vi "Generate_WayPoints_Hopping_CV_RunningAvg.vi"(11 "Input Cluster":T2={"Scan Rate (um/s)"=15.0, "X Start"=15.0, "X End"=15.0, "Y Start"=15.0, "Y End"=15.0, " Z Start"=15.0, "HoppingDistance"=1.0, "V"=15.0, "Z End"=15.0, "Approach Rate Hopping (um/s)"=15.0, "Retrack Rate (um/s)"=15.0, "V 2"=15.0, "Approach Rate (um/s)"=15.0, "V 3"=15.0, "CV Rate / V/s"=15.0, "V 4"=15.0, "V 1"=15.0, "HoldTime1/s"=15.0, "Hold time 2 / s"=15.0, "Hold time 3/ s"=15.0, "V2 (AO4)Approach"=15.0, "V2 (AO4)CV"=15.0}) -> (0 "output cluster":T1)   [LabVIEW 2023]
uses:
  TypeDefs/WayPointCluster.ctl
  User_Vi/Settings.vi
panel:
  in  "WayPointCluster":T1
  out "Y  P":dbl
  out "X  P":dbl
  out "HoppingDistanceX":dbl
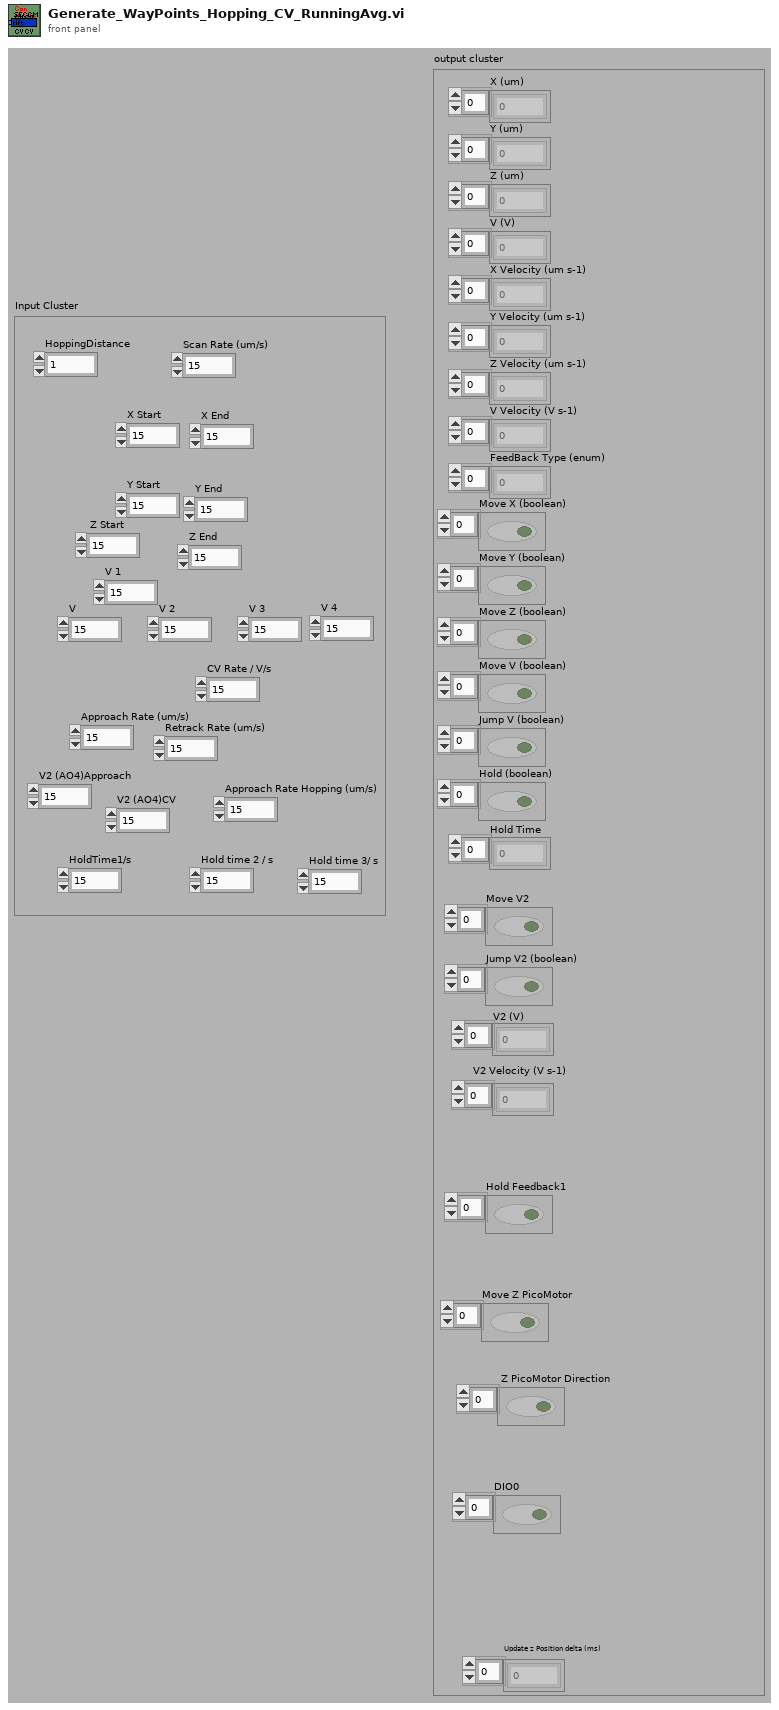
[diagram p1: front panel]
types:
  T1 = typedef "WayPointCluster.ctl" = cluster{"X (um)":dbl[], "Y (um)":dbl[], "Z (um)":dbl[], "V (V)":dbl[], "X Velocity (um s-1)":dbl[], "Y Velocity (um s-1)":dbl[], "Z Velocity (um s-1)":dbl[], "V Velocity (V s-1)":dbl[], "FeedBack Type (enum)":u16[], "Move X (boolean)":bool[], "Move Y (boolean)":bool[], "Move Z (boolean)":bool[], "Move V (boolean)":bool[], "Jump V (boolean)":bool[], "Hold (boolean)":bool[], "Hold Time":u32[], "V2 (V)":dbl[], "Move V2":bool[], "V2 Velocity (V s-1)":dbl[], "Jump V2 (boolean)":bool[], "Update z Position delta (ms)":i16[], "Hold Feedback1":bool[], "Move Z PicoMotor":bool[], " Z PicoMotor Direction":bool[], "DIO0":bool[]}
  T2 = cluster{"Scan Rate (um/s)":dbl, "X Start":dbl, "X End":dbl, "Y Start":dbl, "Y End":dbl, " Z Start":dbl, "HoppingDistance":dbl, "V":dbl, "Z End":dbl, "Approach Rate Hopping (um/s)":dbl, "Retrack Rate (um/s)":dbl, "V 2":dbl, "Approach Rate (um/s)":dbl, "V 3":dbl, "CV Rate / V/s":dbl, "V 4":dbl, "V 1":dbl, "HoldTime1/s":dbl, "Hold time 2 / s":dbl, "Hold time 3/ s":dbl, "V2 (AO4)Approach":dbl, "V2 (AO4)CV":dbl}
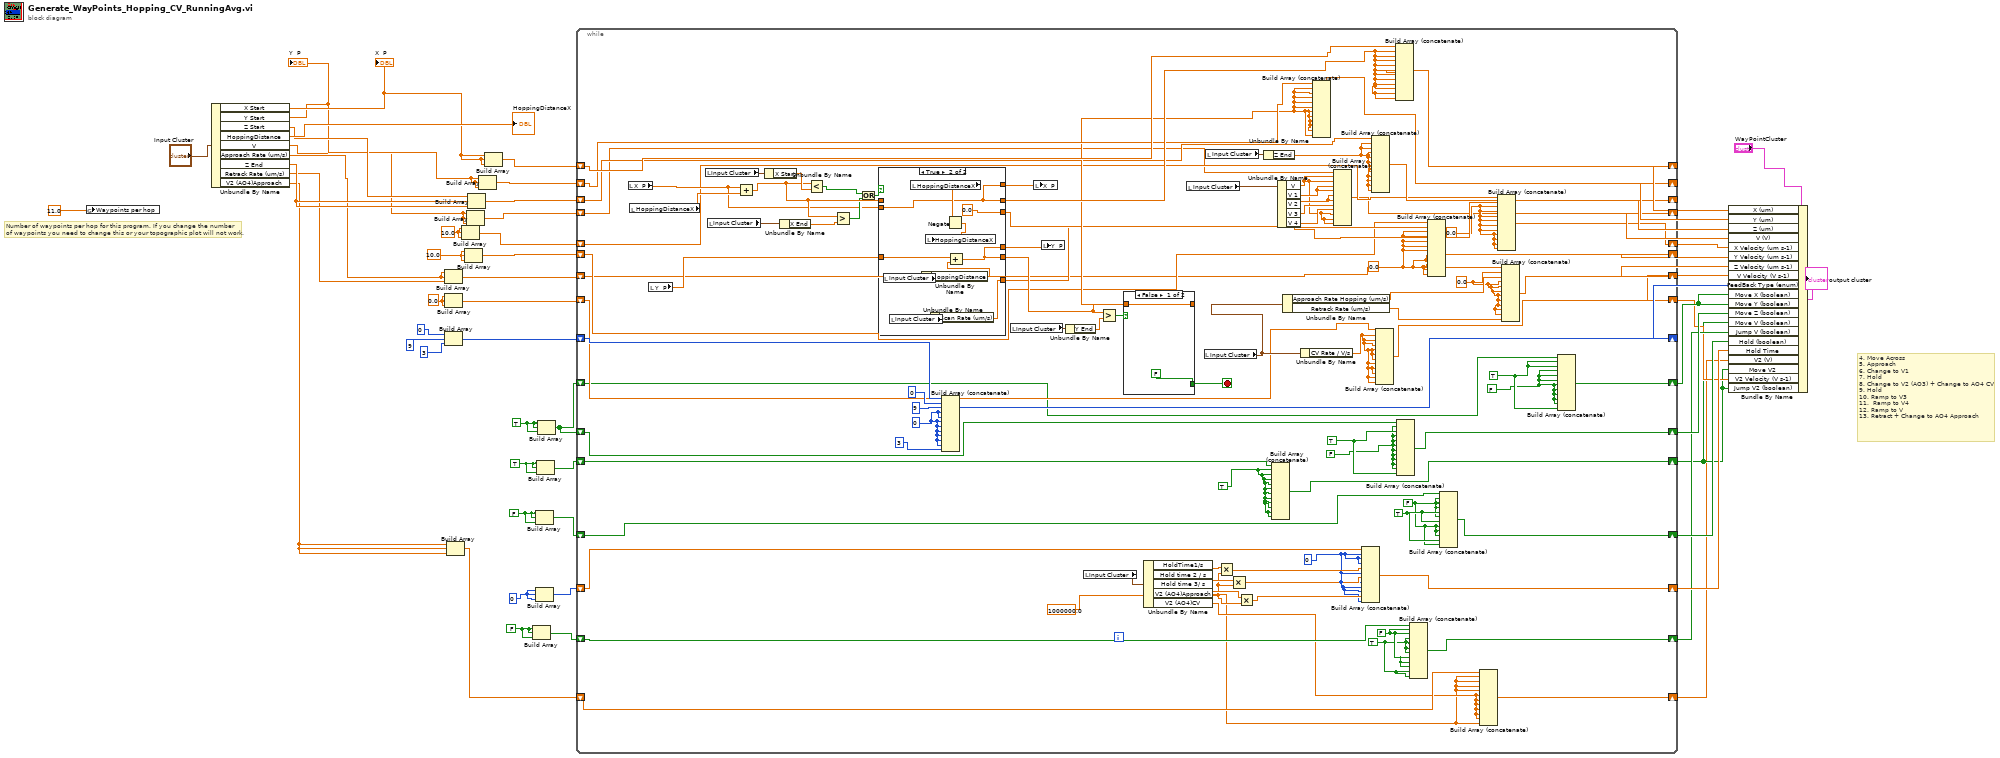
[diagram p0: block diagram]
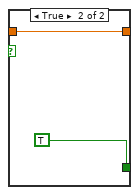
[diagram p2: hidden frame]
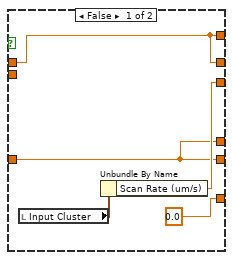
[diagram p3: hidden frame]
diagram:
  w17 = FALSE
  w20 = FALSE
  w19 = u32 0 ("element")
  w18 = TRUE
  w15 = TRUE
  w11 = 10.0 ("element")
  w12 = 10.0 ("element")
  w14 = 0.0 ("element")
  # "Number of waypoints per hop for this program. If you change the number\nof waypoints you need to change this or your topographic plot will not work."
  # "4. Move Across\n5. Approach\n6. Change to V1\n7. Hold\n8. Change to V2 (AO3) + Change to AO4 CV\n9. Hold\n10. Ramp to V3\n11.  Ramp to V4\n12. Ramp to V\n13. Retract + Change to AO4 Approach"
  n1 = global write "Settings.vi" "Waypoints per hop"(11.0) -> ()
  n2 = Unbundle By Name("Input Cluster") -> ("X Start"=w35:dbl, "Y Start"=w34:dbl, "Z Start"=w36:dbl, "HoppingDistance"=→"HoppingDistanceX":dbl, "V"=w32:dbl, "Approach Rate (um/s)"=w13:dbl, "Z End"=w33:dbl, "Retrack Rate (um/s)"=w31:dbl, "V2 (AO4)Approach"=w4:dbl)
  "X  P" <- w35
  "Y  P" <- w34
  n3 = Build Array(w13, w13, w31) -> (w42:dbl[])
  n4 = Build Array(u16 0 ("element"), u16 9 ("element"), u16 3 ("element")) -> (w39:u16[])
  n5 = Build Array(w14, w14, w14) -> (w40:dbl[])
  n6 = Build Array(w4, w4, w4) -> (w3:dbl[])
  n7 = Build Array(w11, w11, w11) -> (w45:dbl[])
  n8 = Build Array(w12, w12, w12) -> (w44:dbl[])
  n9 = Build Array(w32, w32, w32) -> (w47:dbl[])
  n10 = Build Array(w36, w33, w33) -> (w49:dbl[])
  n11 = Build Array(w34, w34, w34) -> (w51:dbl[])
  n12 = Build Array(w35, w35, w35) -> (w53:dbl[])
  n13 = Build Array(w20, w20, w20) -> (w24:bool[])
  n14 = Build Array(w17, w17, w17) -> (w16:bool[])
  n15 = Build Array(w19, w19, w19) -> (w28:u32[])
  n16 = Build Array(w18, w18, w18) -> (w22:bool[])
  n17 = Build Array(w15, w15, w15) -> (w7:bool[])
  n18 = while {
    shift-right: [w120] -> w52
    shift-left: w53 -> [w121]
    shift-right: [w117] -> w50
    shift-left: w51 -> [w118]
    shift-right: [w114] -> w48
    shift-left: w49 -> [w115]
    shift-right: [w104] -> w46
    shift-left: w47 -> [w105]
    shift-right: [w98] -> w29
    shift-left: w45 -> [w112]
    shift-right: [w107] -> w43
    shift-left: w44 -> [w108]
    shift-right: [w96] -> w41
    shift-left: w42 -> [w97]
    shift-right: [w91] -> w6
    shift-left: w40 -> [w92]
    shift-right: [w144] -> w38
    shift-left: w39 -> [w145]
    shift-right: [w88] -> w27
    shift-left: w7 -> [w89]
    shift-right: [w82] -> w26
    shift-left: w16 -> [w83]
    shift-right: [w78] -> w25
    shift-left: w28 -> [w79]
    shift-right: [w68] -> w23
    shift-left: w24 -> [w69]
    shift-right: [w85] -> w5
    shift-left: w22 -> [w86]
    shift-right: [w61] -> w8
    shift-left: w7 -> [w60]
    shift-right: [w58] -> w2
    shift-left: w3 -> [w59]
    stop <- w132 stop-if-true
    w63 = FALSE
    w64 = TRUE
    w65 = 1000000.0 ("y")
    w66 = TRUE
    w110 = 0.0 ("element")
    w84 = TRUE
    w67 = FALSE
    w70 = u32 0 ("element")
    w81 = TRUE
    w80 = FALSE
    w62 = FALSE
    w87 = TRUE
    w123 = u16 0 ("element")
    w106 = 0.0 ("element")
    w94 = 0.0 ("element")
    n19 = local read "X  P"() -> (w131:dbl)
    n20 = local read "HoppingDistanceX"() -> (w146:dbl)
    n21 = local read "Y  P"() -> (w130:dbl)
    n22 = local read "Input Cluster"() -> (w148:T2)
    n23 = local read "Input Cluster"() -> (w147:T2)
    n24 = Add(x=w131, y=w146) -> (x+y=w138:dbl)
    n25 = Unbundle By Name(w148) -> ("X Start"=w141:dbl)
    n26 = Unbundle By Name(w147) -> ("X End"=w139:dbl)
    n27 = Less?(x=w138, y=w141) -> (x < y?=w140:bool)
    n28 = Greater?(x=w138, y=w139) -> (0:w137:bool)
    n29 = Or(x=w140, y=w137) -> (x .or. y?=w136:bool)
    n30 = case shown="True" w136 {
      tunnel: w138 -> [w153 _]
      tunnel: [w153 w159] -> w119
      tunnel: w131 -> [_ w159]
      tunnel: w130 -> [w154 w160]
      tunnel: [w154 w158] -> w129
      tunnel: [w156 0.0] -> w111
      tunnel: [0.0 w161] -> w109
      tunnel: [w154 w158] -> w128
      tunnel: [w153 w159] -> w127
      frame False {
        n31 = local read "Input Cluster"() -> (w157:T2)
        n32 = Unbundle By Name(w157) -> ("Scan Rate (um/s)"=w156:dbl)
      }
      frame True {
        n33 = local read "Input Cluster"() -> (w165:T2)
        n34 = local read "Input Cluster"() -> (w163:T2)
        n35 = local read "HoppingDistanceX"() -> (w167:dbl)
        n36 = Unbundle By Name(w165) -> ("HoppingDistance"=w164:dbl)
        n37 = Unbundle By Name(w163) -> ("Scan Rate (um/s)"=w161:dbl)
        n38 = Negate(x=w167) -> (-x=w166:dbl)
        n39 = local write "HoppingDistanceX"(w166) -> ()
        n40 = Add(x=w160, y=w164) -> (x+y=w158:dbl)
      }
    }
    n41 = Build Array (concatenate)(w145, u16 0 ("element"), u16 9 ("element"), w123, w123, w123, w123, w123, w123, w123, w123, u16 3 ("element")) -> (w144:u16[])
    n42 = local read "Input Cluster"() -> (w135:T2)
    n43 = local write "X  P"(w127) -> ()
    n44 = local write "Y  P"(w128) -> ()
    n45 = Unbundle By Name(w135) -> ("Y End"=w134:dbl)
    n46 = local read "Input Cluster"() -> (w77:T2)
    n47 = Greater?(x=w129, y=w134) -> (0:w133:bool)
    n48 = case shown="False" w133 {
      tunnel: w129 -> [w150 w152]
      tunnel: [w150 w152] -> w116
      tunnel: [FALSE TRUE] -> w132
      frame False {
      }
      frame True {
      }
    }
    n49 = Unbundle By Name(w77) -> ("HoldTime1/s"=w76:dbl, "Hold time 2 / s"=w75:dbl, "Hold time 3/ s"=w74:dbl, "V2 (AO4)Approach"=w56:dbl, "V2 (AO4)CV"=w57:dbl)
    n50 = local read "Input Cluster"() -> (w142:T2)
    n51 = local read "Input Cluster"() -> (w124:T2)
    n52 = local read "Input Cluster"() -> (w143:T2)
    n53 = Multiply(x=w76, y=w65) -> (x*y=w73:dbl)
    n54 = Multiply(x=w75, y=w65) -> (x*y=w72:dbl)
    n55 = Multiply(x=w74, y=w65) -> (x*y=w71:dbl)
    n56 = Unbundle By Name(w143) -> ("Z End"=w113:dbl)
    n57 = Build Array (concatenate)(w86, w84, w84, w84, w84, w84, w84, w84, w84, w84, w84, w84) -> (w85:bool[])
    n58 = Unbundle By Name(w142) -> ("V"=w99:dbl, "V 1"=w103:dbl, "V 2"=w102:dbl, "V 3"=w101:dbl, "V 4"=w100:dbl)
    n59 = Unbundle By Name(w124) -> ("Approach Rate Hopping (um/s)"=w95:dbl, "Retrack Rate (um/s)"=w93:dbl)
    n60 = Unbundle By Name(w124) -> ("CV Rate / V/s"=w90:dbl)
    n61 = Build Array (concatenate)(w118, w116, w116, w116, w116, w116, w116, w116, w116, w116, w116, w116) -> (w117:dbl[])
    n62 = Build Array (concatenate)(w105, w99, w99, w103, w103, w102, w102, w101, w100, w99, w99, w99) -> (w104:dbl[])
    n63 = Build Array (concatenate)(w79, w70, w70, w70, w73, w70, w72, w70, w70, w70, w71, w70) -> (w78:dbl[])
    n64 = Build Array (concatenate)(w115, w113, w113, w113, w113, w113, w113, w113, w113, w113, w113, w113) -> (w114:dbl[])
    n65 = Build Array (concatenate)(w92, w90, w90, w90, w90, w90, w90, w90, w90, w90, w90, w90) -> (w91:dbl[])
    n66 = Build Array (concatenate)(w121, w119, w119, w119, w119, w119, w119, w119, w119, w119, w119, w119) -> (w120:dbl[])
    n67 = Build Array (concatenate)(w89, w62, w87, w62, w62, w62, w62, w62, w62, w62, w62, w87) -> (w88:bool[])
    n68 = Build Array (concatenate)(w69, w67, w67, w66, w66, w66, w66, w67, w67, w67, w66, w66) -> (w68:bool[])
    n69 = Build Array (concatenate)(w108, w109, w106, w106, w106, w106, w106, w106, w106, w106, w106, w106) -> (w107:dbl[])
    n70 = Build Array (concatenate)(w83, w80, w80, w80, w81, w80, w81, w80, w80, w80, w81, w80) -> (w82:bool[])
    n71 = Build Array (concatenate)(w59, w56, w56, w56, w56, w57, w57, w57, w57, w57, w57, w56) -> (w58:dbl[])
    n72 = Build Array (concatenate)(w112, w111, w110, w110, w110, w110, w110, w110, w110, w110, w110, w110) -> (w98:dbl[])
    n73 = Build Array (concatenate)(w97, w94, w95, w94, w94, w94, w94, w94, w94, w94, w94, w93) -> (w96:dbl[])
    n74 = Build Array (concatenate)(w60, w64, w64, w63, w63, w63, w63, w63, w63, w63, w63, w64) -> (w61:bool[])
  }
  n75 = Bundle By Name(cluster="WayPointCluster", "X (um)"=w52, "Y (um)"=w50, "Z (um)"=w48, "V (V)"=w46, "X Velocity (um s-1)"=w29, "Y Velocity (um s-1)"=w43, "Z Velocity (um s-1)"=w41, "V Velocity (V s-1)"=w6, "FeedBack Type (enum)"=w38, "Move X (boolean)"=w8, "Move Y (boolean)"=w8, "Move Z (boolean)"=w27, "Move V (boolean)"=w5, "Jump V (boolean)"=w23, "Hold (boolean)"=w26, "Hold Time"=w25, "V2 (V)"=w2, "Move V2"=w5, "V2 Velocity (V s-1)"=w6, "Jump V2 (boolean)"=w5) -> (→"output cluster":T1)
